vi "ControlSetConfig.vi"(0 "Task ID":u32, 1 "error in (no error)":errorcluster) -> (3 "Task ID":u32, 5 "error out":errorcluster)   [LabVIEW 2015]
uses:
  Windows/System32/AdvLvDaq.dll
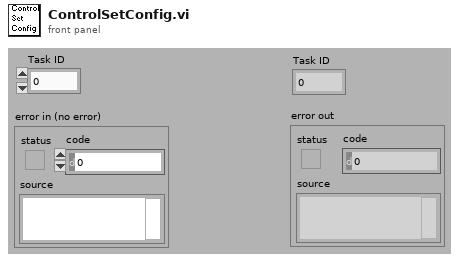
[diagram p1: front panel]
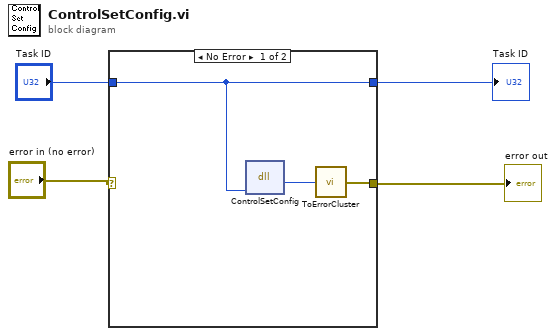
[diagram p0: block diagram]
diagram:
  n1 = case shown="No Error" "error in (no error)" {
    selector: "error in (no error)" -> [_ w9]
    tunnel: "Task ID" -> [w5 w8]
    tunnel: [w7 w9] -> w2
    tunnel: [w5 w8] -> w1
    frame No Error {
      n2 = dll-call lib="C:/Windows/System32/AdvLvDaq.dll" fn="ControlSetConfig"("taskId"=w5) -> ("return type"=w6:i32)  [unwired: 4 in, 2 out]
      n3 = call "ToErrorCluster.vi"("error code"=w6) -> ("error out"=w7:errorcluster)
    }
    frame Error {
    }
  }
  "error out" <- w2
  "Task ID" <- w1
